vi "Run.vi"(9 "Team In":refnum<class "Team.lvclass">, 11 "MySquare in":refnum<class "MySquare.lvclass">) -> (1 "Team":refnum<class "Team.lvclass">, 2 "Run Result":T1, 3 "MySquare out":refnum<class "MySquare.lvclass">)   [LabVIEW 2020, in "Galaxy.lvlib" / "MySquare.lvclass"]
doc: "This VI is called on every active square each turn of the game for the square to decide what action to take."
uses:
  MySquare.lvclass
  C:/dev/sol-squarebattle/SquareBattle/Square/Square.lvclass
  SquareBattle/Run Result.ctl
  SquareBattle/Square/Square.lvclass
  SquareBattle/Action.ctl
  SquareBattle/Direction.ctl
  SquareBattle/Team/Team.lvclass
  MyTeam/MyTeam.lvclass
  C:/dev/sol-squarebattle/SquareBattle/Team/Team.lvclass
  SquareBattle/SquareBattle.lvlib
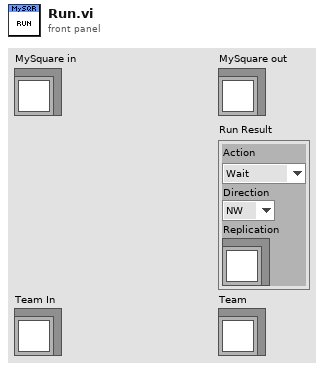
[diagram p1: front panel]
types:
  T1 = typedef "SquareBattle.lvlib/Run Result.ctl" = cluster{"Action":T2, "Direction":T3, "Replication":refnum<class "Square.lvclass">}
  T2 = typedef "SquareBattle.lvlib/Action.ctl" = enum16{"Wait", "Move", "Attack", "Replicate"}
  T3 = typedef "SquareBattle.lvlib/Direction.ctl" = enum16{"NW", "N", "NE", "E", "SE", "S", "SW", "W"}
  T4 = typedef "SquareBattle.lvlib/Location Status.ctl" = cluster{"Empty":bool, "Friend":bool, "Enemy":bool}
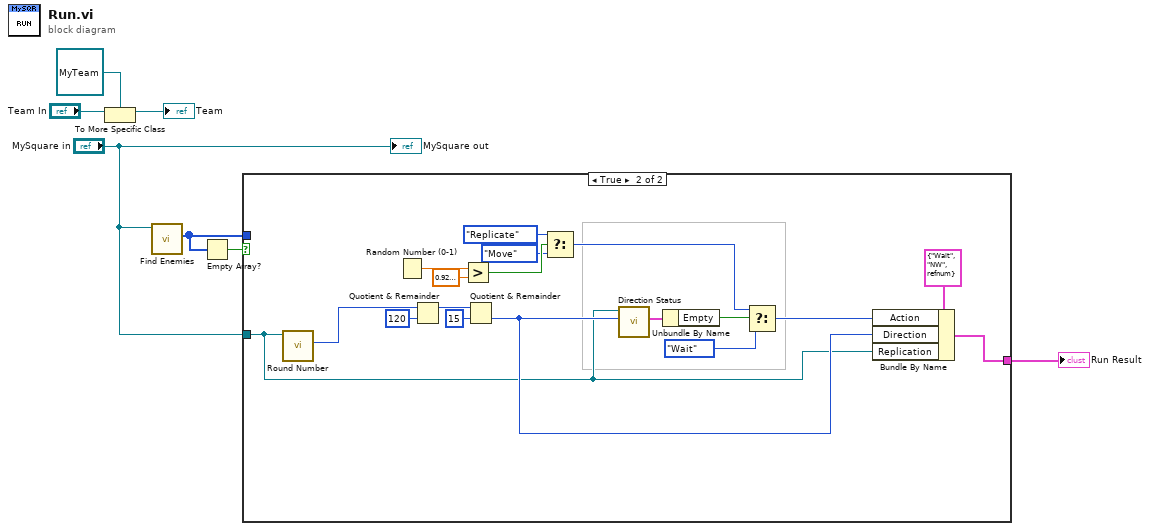
[diagram p0: block diagram]
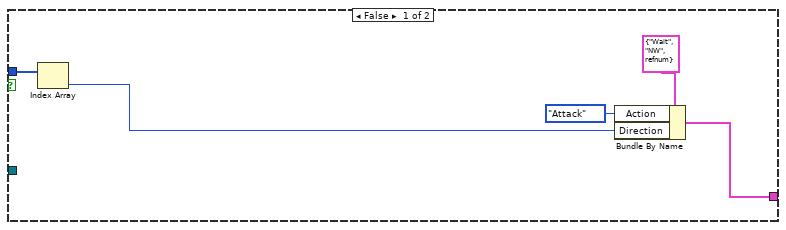
[diagram p2: hidden frame]
diagram:
  n1 = To More Specific Class(target class=refnum<class "MyTeam.lvclass"> refnum ("SquareTeam.lvlib:MyTeam.lvclass"), reference="Team In") -> (specific class reference=→"Team":refnum<class "MyTeam.lvclass">)  [unwired: 1 in, 1 out]
  n2 = call "Find Enemies.vi"("Square"="MySquare in") -> ("Enemy Directions"=w3:T3[])  [unwired: 9 in, 1 out]
  n3 = Empty Array?(array=w3) -> (empty?=w4:bool)
  n4 = case shown="True" w4 {
    tunnel: w3 -> [w12 _]
    tunnel: [w8 w13] -> w2
    tunnel: "MySquare in" -> [_ w14]
    frame False {
      n5 = Index Array(array=w12) -> (element=w9:T3)  [unwired: 1 in]
      n6 = Bundle By Name(cluster=T1 {"Action"=enum."Wait", "Direction"=enum."NW", "Replication"=refnum} ("Run Result"), "Action"=Action."Attack", "Direction"=w9) -> (w8:T1)
    }
    frame True {
      n7 = call "Round Number.vi"("Square in"=w14) -> ("Round Number"=w22:u32)  [unwired: 10 in]
      n8 = Random Number (0-1)() -> (number: 0 to 1=w30:dbl)
      n9 = Quotient & Remainder(x=w22, y=120) -> (x-y*floor(x/y)=w23:u32)  [unwired: 1 out]
      n10 = Greater?(x=w30, y=0.9299999999999999) -> (0:w28:bool)
      n11 = Quotient & Remainder(x=w23, y=15) -> (floor(x/y)=w15:u32)  [unwired: 1 out]
      n12 = Select(t=enum16{"Wait", "Move", "Attack", "Replicate"}."Replicate" ("Action"), s=w28, f=enum16{"Wait", "Move", "Attack", "Replicate"}."Move" ("Action")) -> (s? t:f=w19:enum16{"Wait", "Move", "Attack", "Replicate"})
      n13 = call "Direction Status.vi"("Direction"=w15, "Square"=w14) -> ("Status"=w21:T4)  [unwired: 9 in]
      n14 = Unbundle By Name(w21) -> ("Empty"=w20:bool)
      n15 = Select(t=w19, s=w20, f=enum16{"Wait", "Move", "Attack", "Replicate"}."Wait") -> (s? t:f=w16:enum16{"Wait", "Move", "Attack", "Replicate"})
      n16 = Bundle By Name(cluster=T1 {"Action"=enum."Wait", "Direction"=enum."NW", "Replication"=refnum} ("Run Result"), "Action"=w16, "Direction"=w15, "Replication"=w14) -> (w13:T1)
    }
  }
  "Run Result" <- w2
  "MySquare out" <- "MySquare in"
